vi "Find Potential Tips.vi"(4 "dy":i32, 6 "dx":i32, 7 "Frame Number":i32, 8 "error in (no error)":errorcluster, 9 "ROI Height":i32, 10 "ROI Width":i32, 11 "Image":T4) -> (0 "error out":errorcluster, 2 "Potential Tips":T1[](array[typedef]) {"ROI Descriptor"."Contours"."Type" items=["No Selection", "Point", "Line", "Rectangle", "Oval", "Polygon", "Freehand Region", "Annulus", "Unused2", "Unused3", "Broken Line", "Freehand Line", "Rotated Rectangle"]; "Point"."Y" format="%.2f"; "Point"."X" format="%.2f"}, 3 "Image out":T4)   [LabVIEW 2013]
uses:
  <vilib>/vision/Image Controls.llb/IMAQ Image.ctl
  Controls/Tip.ctl
  <vilib>/vision/NI_Vision_Development_Module.lvlib
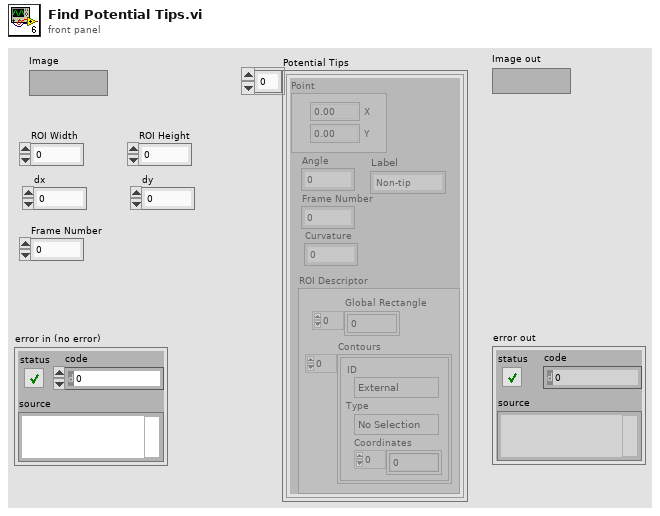
[diagram p1: front panel]
types:
  T1 = typedef "Tip.ctl" = cluster{"Point":T2, "Angle":dbl, "Frame Number":i32, "ROI Descriptor":T3, "Curvature":dbl, "Label":string}
  T2 = typedef "IMAQ Point" = cluster{"X":sgl, "Y":sgl}
  T3 = typedef "ROI Descriptor" = cluster{"Global Rectangle":i32[], "Contours":cluster{"ID":enum32{"External", "Internal"}, "Type":u32, "Coordinates":i32[]}[]}
  T4 = typedef "IMAQ Image.ctl" = refnum<image>
  T5 = enum32{"AutoM", "Close", "Dilate", "Erode", "Gradient", "Gradient out", "Gradient in", "Hit miss", "Open", "PClose", "POpen", "Thick", "Thin"}
  T6 = typedef "IMAQ Rectangle" = cluster{"Left":i32, "Top":i32, "Right":i32, "Bottom":i32, "Rotation":dbl}
  T7 = typedef "Image Type" = u32
  T8 = enum16{"Rect Left To Right", "Rect Right To Left", "Rect Top To Bottom", "Rect Bottom To Top", "Annulus Inner To Outer", "Annulus Outer To Inner", "Annulus Start Angle To End Angle", "Annulus End Angle To Start Angle"}
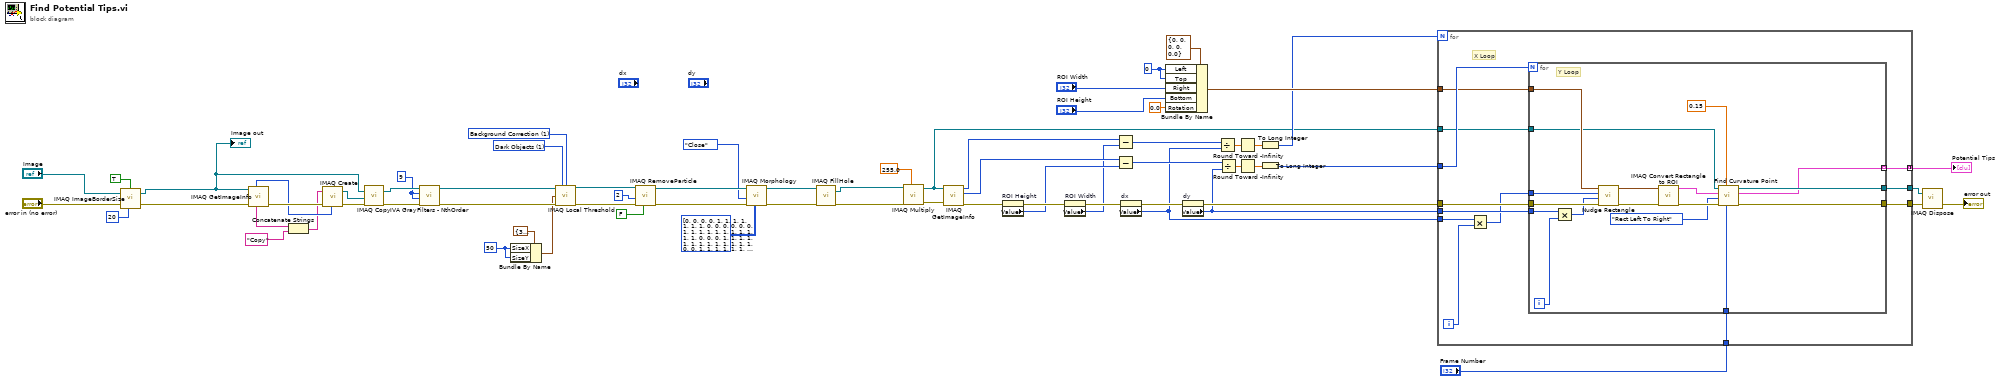
[diagram p0: block diagram]
diagram:
  w15 = 50 ("SizeX")
  w18 = u32 1 items=["Bright Objects", "Dark Objects"] ("Look For (Bright Objects)")
  w19 = u32 1 items=["Niblack", "Background Correction"] ("Method (Niblack)")
  w57 = 0 ("Left")
  w59 = 9 ("Filter size X")
  n1 = call "IMAQ ImageBorderSize"("Get/Set Status? (Set)"=TRUE, "Image"="Image", "Image border size in"=20 ("Border Size"), "error in (no error)"="error in (no error)") -> ("Image Out"=w20:T4, "error out"=w21:errorcluster)  [unwired: 1 out]
  "Image out" <- w20
  n2 = call "IMAQ GetImageInfo"("error in (no error)"=w21, "Image"=w20) -> ("error out"=w68:errorcluster, "Image Name"=w66:string, "Image Type"=w67:T7)  [unwired: 2 in, 5 out]
  n3 = Concatenate Strings(w66, "Copy" ("string")) -> (w64:string)
  n4 = call "IMAQ Create"("Image Name"=w64, "Image Type"=w67, "error in (no error)"=w68) -> ("New Image"=w62:T4, "error out"=w63:errorcluster)  [unwired: 2 in]
  n5 = call "IMAQ Copy"("error in (no error)"=w63, "Image Dst"=w62, "Image Src"=w20) -> ("error out"=w61:errorcluster, "Image Dst Out"=w60:T4)  [unwired: 3 in]
  n6 = call <vilib>:"IVA GrayFilters - NthOrder.vi"("error in"=w61, "Filter size Y"=w59, "Filter size X"=w59, "Image In"=w60) -> ("error out"=w37:errorcluster, "Image Out"=w38:T4)  [unwired: 6 out]
  n7 = Bundle By Name(cluster=cluster{"SizeX":i32, "SizeY":i32} {"SizeX"=32, "SizeY"=32} ("Window Size (32x32)"), "SizeX"=w15, "SizeY"=w15) -> (w16:cluster{"SizeX":i32, "SizeY":i32})
  n8 = call "IMAQ Local Threshold"("Image Src"=w38, "Look For (Bright Objects)"=w18, "Method (Niblack)"=w19, "Window Size (32x32)"=w16, "error in (no error)"=w37) -> ("Image Dst Out"=w6:T4, "error out"=w5:errorcluster)  [unwired: 9 in]
  n9 = call "IMAQ RemoveParticle"("Low Pass/High Pass (Low)"=FALSE, "error in (no error)"=w5, "Number of Erosion"=2, "Image Src"=w6) -> ("error out"=w12:errorcluster, "Image Dst Out"=w11:T4)  [unwired: 3 in, 3 out]
  n10 = call "IMAQ Morphology"("Structuring Element"=i32[][] [[0, 0, 0, 0, 1, 1, 1, 1, 1, 1, 1, 0, 0, 0, 0], [0, 0, 1, 1, 1, 1, 1, 1, 1, 1, 1, 1, 1, 0, 0], [0, 1, 1, 1, 1, 1, 1, 1, 1, 1, 1, 1, 1, 1, 0], [0, 1, 1, 1, 1, 1, 1, 1, 1, 1, 1, 1, 1, 1, 0], [1, 1, 1, 1, 1, 1, 1, 1, 1, 1, 1, 1, 1, 1, 1], [1, 1, 1, 1, 1, 1, 1, 1, 1, 1, 1, 1, 1, 1, 1], [1, 1, 1, 1, 1, 1, 1, 1, 1, 1, 1, 1, 1, 1, 1], [1, 1, 1, 1, 1, 1, 1, 1, 1, 1, 1, 1, 1, 1, 1], [1, 1, 1, 1, 1, 1, 1, 1, 1, 1, 1, 1, 1, 1, 1], [1, 1, 1, 1, 1, 1, 1, 1, 1, 1, 1, 1, 1, 1, 1], [1, 1, 1, 1, 1, 1, 1, 1, 1, 1, 1, 1, 1, 1, 1], [0, 1, 1, 1, 1, 1, 1, 1, 1, 1, 1, 1, 1, 1, 0], [0, 1, 1, 1, 1, 1, 1, 1, 1, 1, 1, 1, 1, 1, 0], [0, 0, 1, 1, 1, 1, 1, 1, 1, 1, 1, 1, 1, 0, 0], [0, 0, 0, 0, 1, 1, 1, 1, 1, 1, 1, 0, 0, 0, 0]], "error in (no error)"=w12, "Operation"=T5."Close", "Image Src"=w11) -> ("error out"=w8:errorcluster, "Image Dst Out"=w7:T4)  [unwired: 3 in, 3 out]
  n11 = call "IMAQ FillHole"("error in (no error)"=w8, "Image Src"=w7) -> ("error out"=w3:errorcluster, "Image Dst Out"=w4:T4)  [unwired: 2 in, 2 out]
  n12 = call "IMAQ Multiply"("Image Src A"=w4, "Constant"=sgl 255.0, "error in (no error)"=w3) -> ("Image Dst Out"=w28:T4, "error out"=w36:errorcluster)  [unwired: 4 in]
  n13 = call "IMAQ GetImageInfo"("error in (no error)"=w36, "Image"=w28) -> ("error out"=w50:errorcluster, "Y Resolution"=w47:i32, "X Resolution"=w48:i32)  [unwired: 2 in, 5 out]
  n14 = property on="ROI Height" class="DigNum (strict)"(error in=w50) -> (error out=w55:errorcluster, "Value"=w46:i32)  [unwired: 1 in, 1 out]
  n15 = property on="ROI Width" class="DigNum (strict)"(error in=w55) -> (error out=w49:errorcluster, "Value"=w45:i32)  [unwired: 1 in, 1 out]
  n16 = Subtract(x=w48, y=w45) -> (x-y=w44:i32)
  n17 = Subtract(x=w47, y=w46) -> (x-y=w43:i32)
  n18 = property on="dx" class="DigNum (strict)"(error in=w49) -> (error out=w42:errorcluster, "Value"=w31:i32)  [unwired: 1 in, 1 out]
  n19 = Bundle By Name(cluster=T6 {"Left"=0, "Top"=0, "Right"=0, "Bottom"=0, "Rotation"=0.0} ("Rectangle"), "Left"=w57, "Top"=w57, "Right"="ROI Width", "Bottom"="ROI Height", "Rotation"=0.0) -> (w33:T6)
  n20 = property on="dy" class="DigNum (strict)"(error in=w42) -> (error out=w32:errorcluster, "Value"=w30:i32)  [unwired: 1 in, 1 out]
  n21 = Divide(x=w44, y=w31) -> (x/y=w54:dbl)
  n22 = Divide(x=w43, y=w30) -> (x/y=w52:dbl)
  n23 = Round Toward -Infinity(1:w54) -> (0:w53:dbl)
  n24 = Round Toward -Infinity(1:w52) -> (0:w51:dbl)
  n25 = To Long Integer(number=w53) -> (32bit integer=w29:i32)
  n26 = To Long Integer(number=w51) -> (32bit integer=w34:i32)
  n27 = for {
    N: w29 -> [_]
    tunnel: w34 -> [w80]
    tunnel: w31 -> [w79]
    tunnel: w30 -> [w78]
    tunnel: w32 -> [w77]
    tunnel: w33 -> [w76]
    tunnel: [w74] -> w27
    tunnel: [w73] -> w26
    tunnel: [w72] -> w2 mode=concatenating
    tunnel: "Frame Number" -> [w71]
    tunnel: w28 -> [w69]
    i -> [w70]
    # "X Loop"
    n28 = Multiply(x=w79, y=w70) -> (x*y=w75:i32)
    n29 = for {
      N: w80 -> [_]
      tunnel: w78 -> [w97]
      tunnel: w77 -> [w95]
      tunnel: w76 -> [w90]
      tunnel: w75 -> [w93]
      tunnel: [w85] -> w74
      tunnel: [w84] -> w73
      tunnel: [w81] -> w72 mode=indexing
      tunnel: w71 -> [w83]
      tunnel: w69 -> [w82]
      i -> [w96]
      # "Y Loop"
      n30 = Multiply(x=w97, y=w96) -> (x*y=w94:i32)
      n31 = call "Nudge Rectangle.vi"("error in (no error)"=w95, "dy"=w94, "dx"=w93, "Rectangle"=w90) -> ("error out"=w92:errorcluster, "Nudged Rectangle"=w91:T6)  [unwired: 6 in]
      n32 = call "IMAQ Convert Rectangle to ROI"("error in (no error)"=w92, "Rectangle"=w91) -> ("error out"=w89:errorcluster, "ROI Descriptor"=w87:T3)  [unwired: 7 in]
      n33 = call "Find Curvature Point.vi"("Frame Number"=w83, "Min Curvature"=0.15, "error in (no error)"=w89, "Search Direction"=T8."Rect Left To Right", "ROI Descriptor"=w87, "Image"=w82) -> ("error out"=w85:errorcluster, "Tip"=w81:T1, "Image out"=w84:T4)  [unwired: 3 in]
    }
  }
  "Potential Tips" <- w2
  n34 = call "IMAQ Dispose"("Image"=w26, "error in (no error)"=w27) -> ("error out"=→"error out":errorcluster)  [unwired: 4 in]
